vi "NameSurnameID.vi"() -> ()   [LabVIEW 2017]
panel:
  in  "Array - String":string[](array[string])
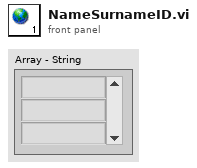
[diagram p1: front panel]
diagram:
